vi "Message Log Shortcut Menu Selection.vi"(6 "ItemPath":string, 8 "error in (no error)":errorcluster, 9 "Coords":T1, 10 "CtlRef":refnum<vi>, 11 "Message Log in":refnum<class "Message Log.lvclass">) -> (0 "error out":errorcluster, 3 "Message Log out":refnum<class "Message Log.lvclass">)   [LabVIEW 2017, in "Message Log.lvclass"]
uses:
  Message Log.lvclass
  <vilib>/Utility/miscctls.llb/LVPoint32TypeDef.ctl
  Listbox Selection.ctl
  <vilib>/Utility/miscctls.llb/LVRowAndColumnTypeDef.ctl
  rql_RCM Filter String.ctl
  rql_RCM Open Running VI.ctl
  rql_RCM Go to Case.ctl
  <vilib>/Utility/error.llb/Error Cluster From Error Code.vi
  <vilib>/ErrorRing/Error Ring.xnode
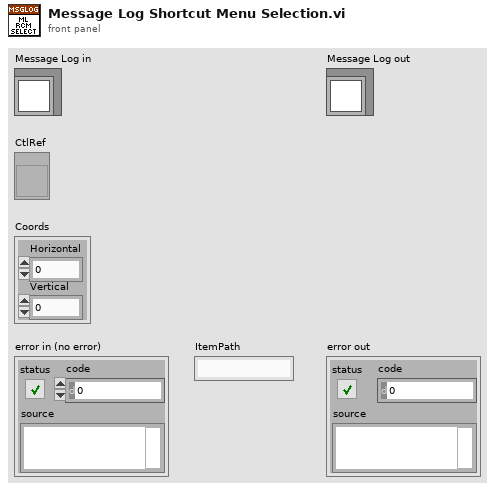
[diagram p1: front panel]
types:
  T1 = typedef "LVPoint32TypeDef.ctl" = cluster{"Horizontal":i32, "Vertical":i32}
  T2 = typedef "Message Log.lvclass/Listbox Selection.ctl" = cluster{"Cell Position":T3, "Row":string[]}
  T3 = typedef "LVRowAndColumnTypeDef.ctl" = cluster{"Row":i32, "Column":i32}
  T4 = typedef "Message Log.lvclass/rql_RCM Filter String.ctl" = cluster{"RCM Listbox Data":T2}
  T5 = typedef "Message Log.lvclass/rql_RCM Open Running VI.ctl" = cluster{"Listbox Selection":T2}
  T6 = typedef "Message Log.lvclass/rql_RCM Go to Case.ctl" = cluster{"Listbox Selection":T2}
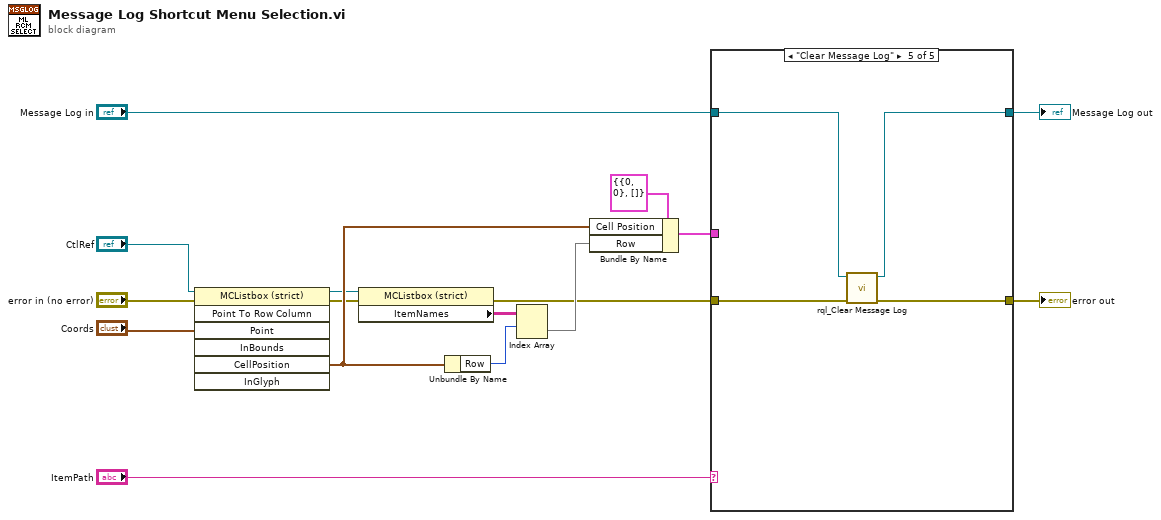
[diagram p0: block diagram]
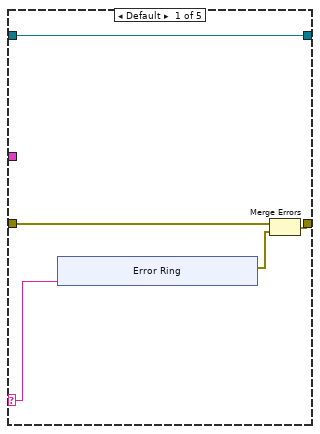
[diagram p2: hidden frame]
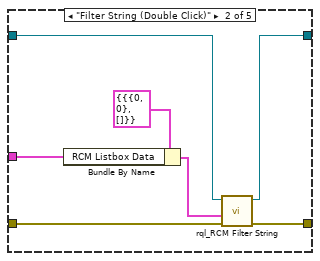
[diagram p3: hidden frame]
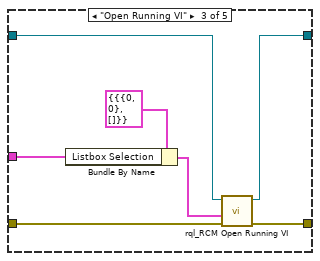
[diagram p4: hidden frame]
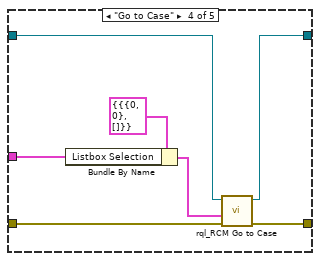
[diagram p5: hidden frame]
diagram:
  n1 = invoke class="MCListbox (strict)" method="Point To Row Column"(reference="CtlRef", error in="error in (no error)", "Point"="Coords") -> (reference out=w13:refnum<vi>, error out=w10:errorcluster, "CellPosition"=w14:T3)  [unwired: 4 in, 4 out]
  n2 = property class="MCListbox (strict)"(reference=w13, error in=w10) -> (error out=w3:errorcluster, "ItemNames"=w11:string[][])  [unwired: 1 out]
  n3 = Unbundle By Name(w14) -> ("Row"=w12:i32)
  n4 = Index Array(array=w11, index (row)=w12) -> (element=w7:string[])  [unwired: 1 in]
  n5 = Bundle By Name(cluster=T2 {"Cell Position"={"Row"=0, "Column"=0}, "Row"=[]} ("Listbox Selection"), "Cell Position"=w14, "Row"=w7) -> (w1:T2)
  n6 = case shown="\"Clear Message Log\"" "ItemPath" {
    selector: "ItemPath" -> [w17 _ _ _ _]
    tunnel: [w21 w32 w39 w46 w50] -> w2
    tunnel: "Message Log in" -> [w21 w33 w40 w47 w51]
    tunnel: [w19 w34 w41 w48 w52] -> w4
    tunnel: w3 -> [w20 w35 w42 w49 w53]
    tunnel: w1 -> [_ w30 w37 w44 _]
    frame Default {
      n7 = xnode "Error Ring"("parameter 0"=w17) -> ("error out"=w18:errorcluster)
      n8 = Merge Errors(w20, w18) -> (w19:errorcluster)
    }
    frame "Filter String (Double Click)" {
      n9 = Bundle By Name(cluster=T4 {"RCM Listbox Data"={"Cell Position"={"Row"=0, "Column"=0}, "Row"=[]}} ("Data"), "RCM Listbox Data"=w30) -> (w29:T4)
      n10 = call "rql_RCM Filter String.vi"("error in"=w35, "Data in"=w29, "Message Log in"=w33) -> ("error out"=w34:errorcluster, "dup Message Log out"=w32:refnum<class "Message Log.lvclass">)  [unwired: 7 in]
    }
    frame "Open Running VI" {
      n11 = Bundle By Name(cluster=T5 {"Listbox Selection"={"Cell Position"={"Row"=0, "Column"=0}, "Row"=[]}} ("Data"), "Listbox Selection"=w37) -> (w36:T5)
      n12 = call "rql_RCM Open Running VI.vi"("error in"=w42, "Data in"=w36, "Message Log in"=w40) -> ("error out"=w41:errorcluster, "dup Message Log out"=w39:refnum<class "Message Log.lvclass">)  [unwired: 7 in]
    }
    frame "Go to Case" {
      n13 = Bundle By Name(cluster=T6 {"Listbox Selection"={"Cell Position"={"Row"=0, "Column"=0}, "Row"=[]}} ("Data"), "Listbox Selection"=w44) -> (w43:T6)
      n14 = call "rql_RCM Go to Case.vi"("error in"=w49, "Data in"=w43, "Message Log in"=w47) -> ("error out"=w48:errorcluster, "dup Message Log out"=w46:refnum<class "Message Log.lvclass">)  [unwired: 7 in]
    }
    frame "Clear Message Log" {
      n15 = call "rql_Clear Message Log.vi"("error in"=w53, "Message Log in"=w51) -> ("error out"=w52:errorcluster, "dup Message Log out"=w50:refnum<class "Message Log.lvclass">)  [unwired: 8 in]
    }
  }
  "Message Log out" <- w2
  "error out" <- w4
